vi "LWXPS_RequestType3.vi"(0 "XPS Reference IN":refnum<k24>, 5 "LabVIEW error IN":errorcluster) -> (12 "XPS Reference OUT":refnum<k24>, 13 "LabVIEW error OUT":errorcluster, 14 "Returned error code":i32, 15 "Header":string, 16 "Time Stamp":string, 17 "Zygo Signal Length 1":string, 18 "Zygo Signal Length 2":string, 19 "XPS Error String":string)   [LabVIEW 2014]
uses:
  D:/XPSQ8_LabView_Library/Development/Source/Dll/Newport.XPS.CommandInterface.dll
  Dll/Newport.XPS.CommandInterface.dll
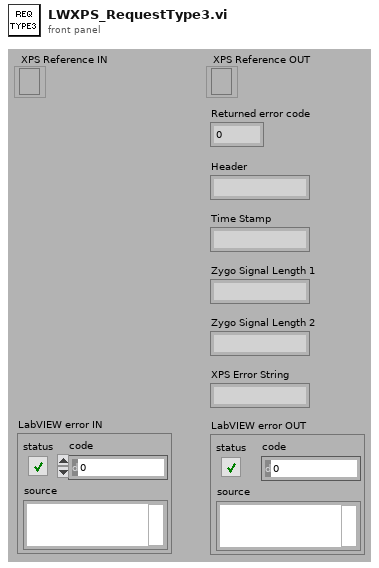
[diagram p1: front panel]
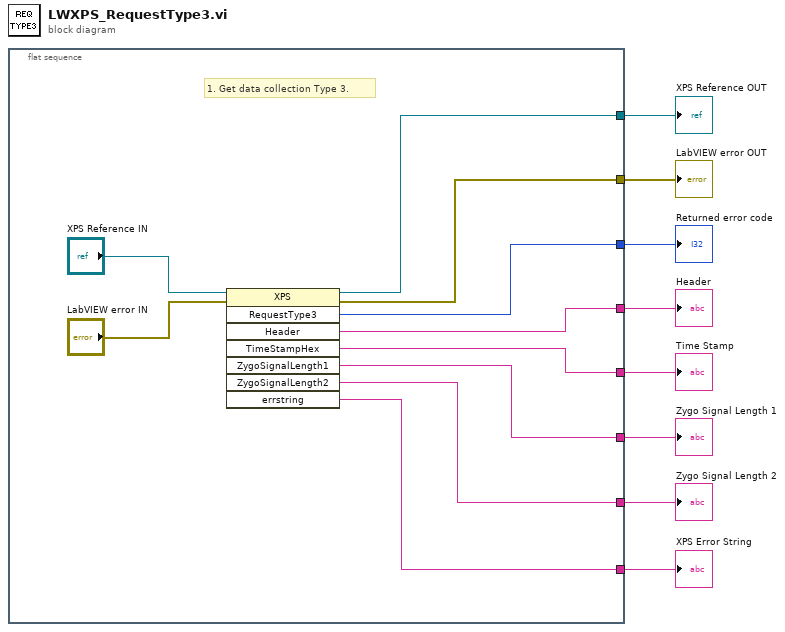
[diagram p0: block diagram]
diagram:
  n1 = flat-sequence {
    tunnel: [w17] -> w8
    tunnel: [w15] -> w7
    tunnel: [w10] -> w6
    tunnel: [w14] -> w5
    tunnel: [w13] -> w3
    tunnel: [w12] -> w1
    tunnel: [w11] -> w4
    tunnel: [w9] -> w2
    frame #0 {
      # "1. Get data collection Type 3."
      n2 = invoke class="XPS" method="RequestType3"(reference="XPS Reference IN", error in="LabVIEW error IN") -> (reference out=w17:refnum<k24>, error out=w15:errorcluster, "RequestType3"=w10:i32, "Header"=w11:string, "TimeStampHex"=w14:string, "ZygoSignalLength1"=w13:string, "ZygoSignalLength2"=w12:string, "errstring"=w9:string)  [unwired: 6 in]
    }
  }
  "XPS Error String" <- w2
  "XPS Reference OUT" <- w8
  "LabVIEW error OUT" <- w7
  "Returned error code" <- w6
  "Time Stamp" <- w5
  "Header" <- w4
  "Zygo Signal Length 1" <- w3
  "Zygo Signal Length 2" <- w1
